vi "Write_Wrap.vi"(8 "error in (no error)":errorcluster, 10 "Value":T1, 11 "Var_DBL in":refnum<class "Var_U16.lvclass">) -> (0 "error out":errorcluster, 3 "Var_DBL out":refnum<class "Var_U16.lvclass">)   [LabVIEW 2021, in "Var_U16.lvclass"]
uses:
  Var_U16.lvclass
  Type.ctl
  Var_U16.lvclass/Var_U16.ctl
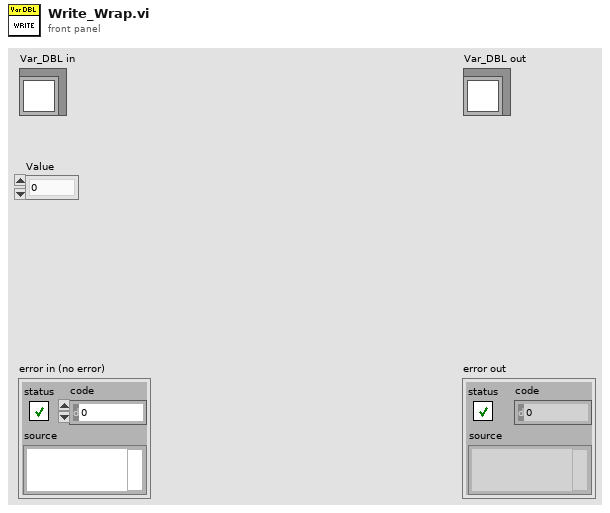
[diagram p1: front panel]
types:
  T1 = typedef "Var_U16.lvclass/Type.ctl" = dbl
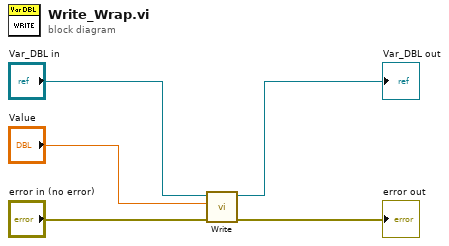
[diagram p0: block diagram]
diagram:
  n1 = call-dynamic "Write.vi"("error in (no error)"="error in (no error)", "Value"="Value", "Double Float.lvclass_340760 in"="Var_DBL in") -> ("error out"=→"error out":errorcluster, "Double Float.lvclass_340760 out"=→"Var_DBL out":refnum<class "Var_U16.lvclass">)  [unwired: 7 in]
